vi "Not A Session - valid session - returns false.vi"() -> ()   [LabVIEW 2013, in "libssh2_tests.lvlib"]
uses:
  libssh2_tests.lvlib
  libssh2/libssh2_init (Default).vi
  <vilib>/addons/_JKI Toolkits/Caraya/classes/Assert/Assert False.vi
  <vilib>/addons/_JKI Toolkits/Caraya/classes/Test/Test.lvclass
  libssh2/libssh2.lvlib
  <vilib>/addons/_JKI Toolkits/Caraya/classes/Assert/Assert.lvclass
panel:
  out "error out":errorcluster
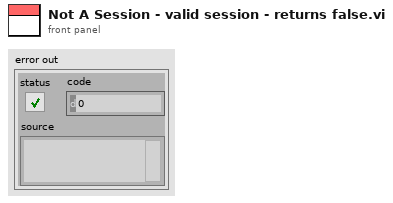
[diagram p1: front panel]
types:
  T1 = typedef "libssh2.lvlib/Session Refnum.ctl" = refnum<k1>
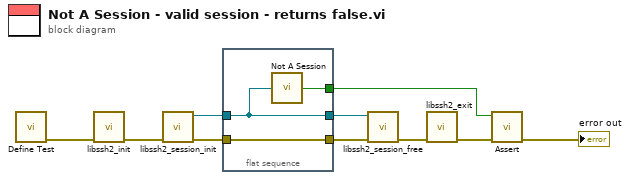
[diagram p0: block diagram]
diagram:
  n1 = call <vilib>:"Define Test.vi"() -> ("error out"=w10:errorcluster)  [unwired: 10 in, 1 out]
  n2 = call-poly "libssh2_init.vi"("error in (no error)"=w10) -> ("error out"=w9:errorcluster)  [unwired: 10 in]
  n3 = call "libssh2_session_init.vi"("error in (no error)"=w9) -> ("error out"=w2:errorcluster, "session"=w4:T1)  [unwired: 9 in]
  n4 = flat-sequence {
    tunnel: [w13] -> w5
    tunnel: w4 -> [w11]
    tunnel: [w12] -> w3
    tunnel: w2 -> [w12]
    tunnel: [w11] -> w1
    frame #0 {
      n5 = call "Not A Session.vi"("session"=w11) -> ("Not a Session?"=w13:bool)
    }
  }
  n6 = call "libssh2_session_free.vi"("error in (no error)"=w3, "session"=w1) -> ("error out"=w7:errorcluster)  [unwired: 9 in]
  n7 = call "libssh2_exit.vi"("error in (no error)"=w7) -> ("error out"=w6:errorcluster)  [unwired: 10 in]
  n8 = call-poly <vilib>:"Assert.vi"("error in (no error)"=w6, "False?"=w5) -> ("error out"=→"error out":errorcluster)  [unwired: 8 in, 1 out]
